vi "Ini_Read_TCPIP.vi"(7 "error in (no error)":errorcluster) -> (0 "error out":errorcluster, 2 "port":u16, 3 "address":string)   [LabVIEW 2020]
doc: "This VI reads the section TCPIP of the PIL.ini file, located at the main directory."
uses:
  <vilib>/Utility/config.llb/Read Key (String).vi
  <vilib>/Utility/config.llb/Read Key (U32).vi
  <vilib>/Utility/config.llb/NI_LVConfig.lvlib
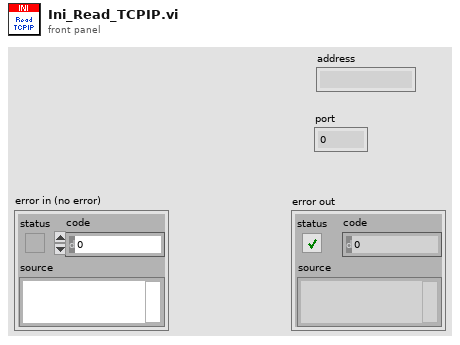
[diagram p1: front panel]
types:
  T1 = typedef "NI_LVConfig.lvlib/Config Data RefNum.ctl" = refnum<k1>
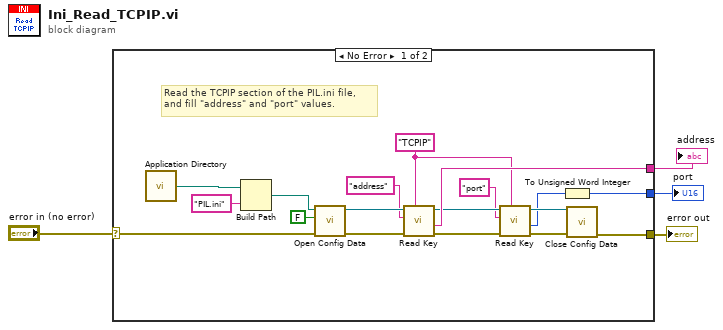
[diagram p0: block diagram]
diagram:
  n1 = case shown="No Error" "error in (no error)" {
    selector: "error in (no error)" -> [w15 w23]
    tunnel: [w14 w23] -> w2
    tunnel: [w5 _] -> w3
    tunnel: [w13 _] -> w1
    frame No Error {
      w10 = "TCPIP" ("section")
      # "Read the TCPIP section of the PIL.ini file,\nand fill \"address\" and \"port\" values."
      n2 = call <vilib>:"Application Directory.vi"() -> ("Application Directory"=w22:path)
      n3 = Build Path(base path=w22, name or relative path="PIL.ini" ("nom ou chemin relatif")) -> (appended path=w21:path)
      n4 = call <vilib>:"Open Config Data.vi"("error in (no error)"=w15, "create file if necessary (T)"=FALSE, "configuration file path"=w21) -> ("error out"=w20:errorcluster, "refnum"=w19:T1)  [unwired: 6 in, 1 out]
      n5 = call-poly <vilib>:"Read Key.vi"("section"=w10, "error in (no error)"=w20, "key"="address", "refnum"=w19) -> ("error out"=w12:errorcluster, "value"=w13:string, "refnum out"=w9:T1)  [unwired: 4 in, 1 out]
      n6 = call-poly <vilib>:"Read Key.vi"("section"=w10, "error in (no error)"=w12, "key"="port", "refnum"=w9) -> ("error out"=w11:errorcluster, "value"=w6:u32, "refnum out"=w8:T1)  [unwired: 4 in, 1 out]
      n7 = To Unsigned Word Integer(number=w6) -> (unsigned 16bit integer=w5:u16)
      n8 = call <vilib>:"Close Config Data.vi"("error in (no error)"=w11, "refnum"=w8) -> ("error out"=w14:errorcluster)  [unwired: 8 in, 1 out]
    }
    frame Error {
    }
  }
  "address" <- w1
  "port" <- w3
  "error out" <- w2
